vi "Add ECU Event Measurement RTM Dependency.vi"(8 "error in (no error)":errorcluster, 9 "Menu hierarchy in":string[](array[string]), 11 "Node Ptr":u64 format="%.0x") -> (0 "error out":errorcluster, 1 "Menu hierarchy out":string[](array[string]), 3 "Action":T1)   [LabVIEW 2011, in "Engine Sim System Explorer.lvlib"]
uses:
  Engine Sim System Explorer.lvlib
  <vilib>/NI Veristand/Custom Device API/Custom Device RTM Dependency.ctl
  Shared/Engine Simulation Global.vi
  <vilib>/NI Veristand/Custom Device API/Get Item Property (Variant).vi
  <vilib>/NI Veristand/Custom Device API/Custom Device API.lvlib
  Engine Simulation Shared.lvlib
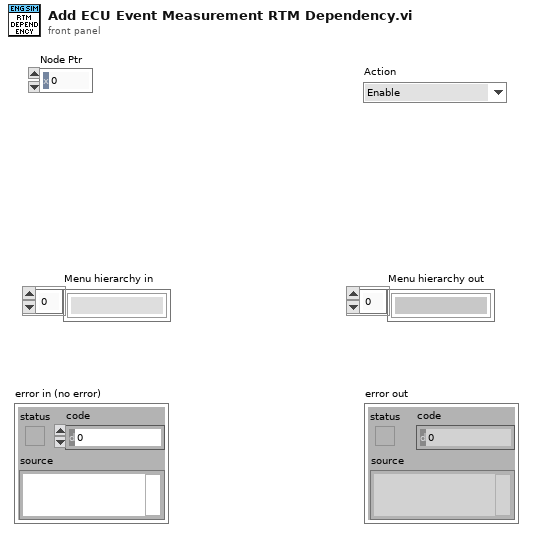
[diagram p1: front panel]
types:
  T1 = typedef "Custom Device API.lvlib/Custom Device RTM Dependency.ctl" = enum16{"Enable", "Disable", "Hide"}
  T2 = cluster{"Time Duration":bool, "Start Angle":bool, "End Angle":bool, "Angle Duration":bool}
  T3 = typedef "Custom Device API.lvlib/Custom Device Item Ref.ctl" = u64
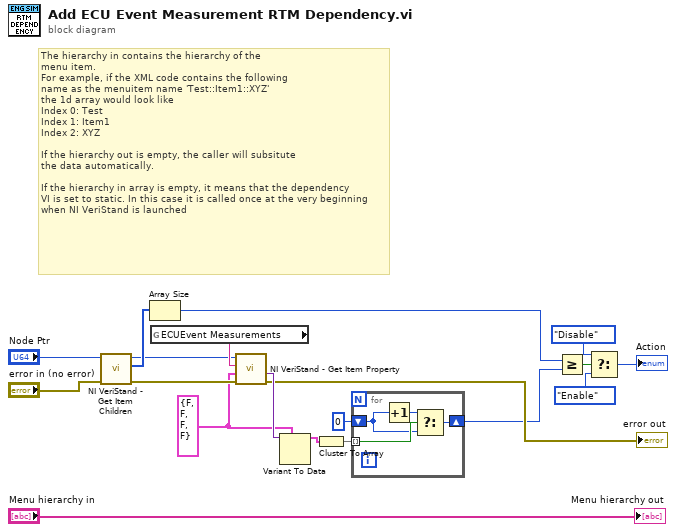
[diagram p0: block diagram]
diagram:
  w4 = T2 {"Time Duration"=FALSE, "Start Angle"=FALSE, "End Angle"=FALSE, "Angle Duration"=FALSE}
  # "The hierarchy in contains the hierarchy of the\nmenu item.\nFor example, if the XML code contains the following\nname as the menuitem name 'Test::Item1::XYZ'\nthe 1d array would look like\nIndex 0: Test\nIndex 1: Item1\nIndex 2: XYZ\n\nIf the hierarchy out is empty, the caller will subsitute\nthe data automatically.\n\nIf the hierarchy in array is empty, it means that the dependency\nVI is set to static. In this case it is called once at the very beginning\nwhen NI VeriStand is launched"
  n1 = call <vilib>:"NI VeriStand - Get Item Children.vi"("error in (no error)"="error in (no error)", "Item Ref in"="Node Ptr") -> ("error out"=w11:errorcluster, "Child Refs"=w17:T3[], "Item Ref out"=w12:T3)  [unwired: 6 in, 1 out]
  n2 = Array Size(array=w17) -> (size(s)=w10:i32)
  n3 = global read "Engine Simulation Global.vi" "ECUEvent Measurements"() -> (w15:string)
  n4 = call-poly <vilib>:"NI VeriStand - Get Item Property.vi"("error in (no error)"=w11, "Default Value"=w4, "Property Name"=w15, "Item Ref in"=w12) -> ("error out"=→"error out":errorcluster, "Value"=w14:variant)  [unwired: 4 in, 2 out]
  n5 = Variant To Data(type=w4, Variant=w14) -> (data=w13:T2)  [unwired: 1 in, 1 out]
  n6 = Cluster To Array(cluster=w13) -> (array=w3:bool[])
  n7 = for {
    tunnel: w3 -> [w22] mode=indexing
    shift-right: [w21] -> w2
    shift-left: 0 -> [w20]
    n8 = Increment(x=w20) -> (x+1=w23:i32)
    n9 = Select(t=w23, s=w22, f=w20) -> (s? t:f=w21:i32)
  }
  n10 = Greater Or Equal?(x=w10, y=w2) -> (x >= y?=w9:bool)
  n11 = Select(t=Custom_Device_RTM_Dependency."Disable" ("Action"), s=w9, f=Custom_Device_RTM_Dependency."Enable" ("Action")) -> (s? t:f=→"Action":T1)
  "Menu hierarchy out" <- "Menu hierarchy in"
